vi "Poly2Dclosed.vi"(11 "Poly2D":T1) -> (3 "Closed":bool)   [LabVIEW 2014]
uses:
  TypeDefs/Poly2D.ctl
  TypeDefs/Point2D.ctl
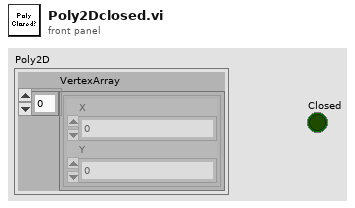
[diagram p1: front panel]
types:
  T1 = typedef "Poly2D.ctl" = cluster{"VertexArray":T2[]}
  T2 = typedef "Point2D.ctl" = cluster{"X":sgl, "Y":sgl}
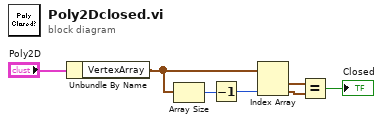
[diagram p0: block diagram]
diagram:
  n1 = Unbundle By Name("Poly2D") -> ("VertexArray"=w1:T2[])
  n2 = Array Size(array=w1) -> (size(s)=w7:i32)
  n3 = Decrement(x=w7) -> (x-1=w6:i32)
  n4 = Index Array(array=w1, index #2=w6) -> (element #1=w5:T2, element #2=w4:T2)  [unwired: 1 in]
  n5 = Equal?(x=w5, y=w4) -> (x = y?=→"Closed":bool)
